vi "Do.vi"(8 "error in (no error)":errorcluster, 10 "Actor in":refnum<class "Actor.lvclass">, 11 "Configure Msg in":refnum<class "Configure Msg.lvclass">) -> (0 "error out":errorcluster, 2 "Actor out":refnum<class "Actor.lvclass">)   [LabVIEW 2016, in "Iterator Actor.lvlib" / "Configure Msg.lvclass"]
doc: "(<B>Filename</B>: Actor Framework.lvlib:Message.lvclass:Do.vi)\n\nDefines what a message does when it is received by an actor. Generally, a message instructs an actor to invoke one of its methods. By default, this method does nothing. A child class must override it to define behavior. Create a child class by using the Actor Framework Message Maker dialog box."
uses:
  Configure Msg.lvclass
  <vilib>/ActorFramework/Actor/Actor.lvclass
  Iterator Actor/Iterator Actor.lvclass
  C:/Program Files (x86)/National Instruments/LabVIEW 2016/vi.lib/ActorFramework/Actor/Actor.lvclass
  Configure Msg.lvclass/Configure Msg.ctl
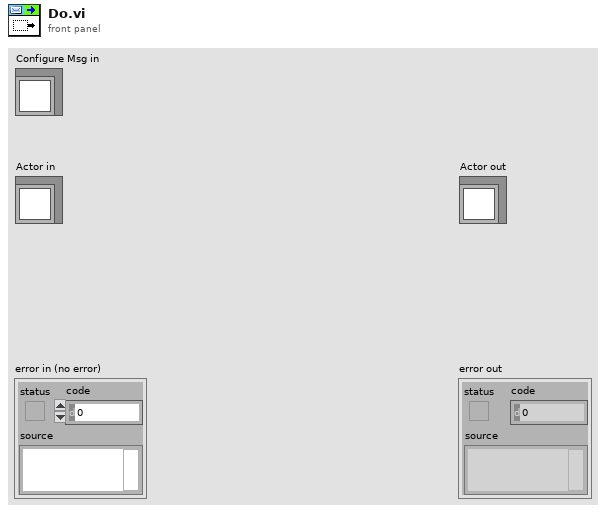
[diagram p1: front panel]
types:
  T1 = typedef "Iterator Actor.lvlib/Iterator Actor.lvclass/Iterator Settings.ctl" = cluster{"Prepare timeout (ms)":i32, "Iterate timeout (ms)":i32, "Conclude timeout (ms)":i32, "Iterate period (ms)":i32, "Number of iterations":i32, "Stop Condition":T2, "Time before stop (ms)":i32, "Prepare Msg":refnum<class "Iterator Reply Msg.lvclass">, "Iterate Msg":refnum<class "Iterator Reply Msg.lvclass">, "Conclude Msg":refnum<class "Iterator Reply Msg.lvclass">, "Error Handler":refnum<class "Iterator Report Error Msg.lvclass">}
  T2 = typedef "Iterator Actor.lvlib/Iterator Actor.lvclass/Stop Condition.ctl" = enum16{"None", "Number of iterations", "Time elapsed", "Iteration result"}
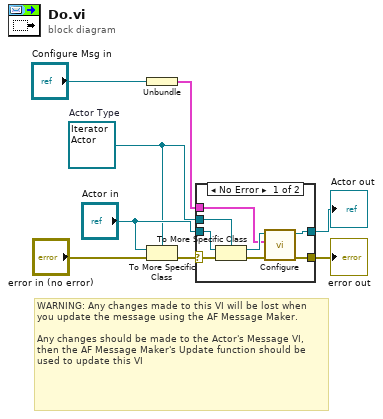
[diagram p0: block diagram]
diagram:
  w3 = refnum<class "Iterator Actor.lvclass"> refnum  # Actor Type
  # "WARNING: Any changes made to this VI will be lost when you update the message using the AF Message Maker.\n\nAny changes should be made to the Actor's Message VI, then the AF Message Maker's Update function should be used to update this VI"
  n1 = Unbundle("Configure Msg in") -> (w2:T1)
  n2 = To More Specific Class(target class=w3, reference="Actor in", error in="error in (no error)") -> (error out=w7:errorcluster)  [unwired: 1 out]
  n3 = case shown="No Error" w7 {
    selector: w7 -> [w16 w18]
    tunnel: [w11 w18] -> w6
    tunnel: [w10 w17] -> w5
    tunnel: "Actor in" -> [w15 w17]
    tunnel: w3 -> [w14 _]
    tunnel: w2 -> [w9 _]
    frame No Error {
      n4 = To More Specific Class ("Actor Cast")(target class=w14, reference=w15, error in=w16) -> (specific class reference=w13:refnum<class "Iterator Actor.lvclass">, error out=w12:errorcluster)
      n5 = call "Configure.vi"("error in (no error)"=w12, "Iterator Settings"=w9, "Iterator Actor in"=w13) -> ("error out"=w11:errorcluster, "Iterator Actor out"=w10:refnum<class "Iterator Actor.lvclass">)  [unwired: 7 in]
    }
    frame Error {
    }
  }
  "error out" <- w6
  "Actor out" <- w5
